vi "host_file_logging.vi"() -> ()   [LabVIEW 2011]
uses:
  Input - Cluster.ctl
  Output - Cluster.ctl
  <vilib>/Platform/TimedLoop/XDataNode/timing_clust.ctl
  <vilib>/Platform/TimedLoop/XDataNode/nitl_modes.ctl
  <vilib>/Platform/TimedLoop/XDataNode/wakeup.ctl
  <vilib>/Platform/TimedLoop/XDataNode/XDataNode.xnode
  <vilib>/Platform/TimedLoop/XDataNode/XDNodeRunTimeDep.lvlib
panel:
  in  "stop":bool
  in  "Pfad":path=path "T:/Projekt_B2G_FABES/B2G/Messprotokolle_B2G1"
  in  "Interval [s]":u32=60 min=1 step=1
  in  "Output - Cluster":T1 {"pHS-1 [pH]" format="%.2g"; "TS-4 [°C]" format="%#.2g"; "FS-2 [l]" format="%.2g"; "FS-1 [l]" format="%.2g"; "DS-1 [bar]" format="%#.2g"; "DFS-1 [l/min]" format="%#.2g"; "FS-3 [l]" format="%.2g"; "DFS-1 [l]" format="%.0g"}
  in  "File Log":bool
  in  "Input - Cluster":T2 {"P-5 AUS [min]" max=100 step=1 format="%#_3g"; "P-5 EIN [min]" step=1 format="%#_3g"; "Hysterese [°C]" format="%.1g"; "P-5 Drehzahl [%]" max=100 step=1 format="%#_3g"; "P-4 Drehzahl [%]" max=100 step=1 format="%#_3g"}
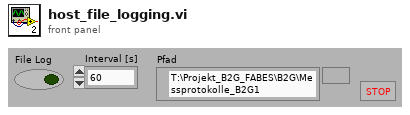
[diagram p1: front panel]
types:
  T1 = typedef "Output - Cluster.ctl" = cluster{"DFS-1 [l]":u64, "FS-3 [l]":dbl, "DFS-1 [l/min]":dbl, "DS-1 [bar]":dbl, "V-10 ZU":bool, "V-14 ZU":bool, "FS-1 [l]":dbl, "FS-2 [l]":dbl, "TS-4 [°C]":dbl, "HS-1":bool, "V-13 [%]":u8, "V-15 [%]":u8, "P-4 [%]":u8, "P-5 [%]":u8, "Dosierung":bool, "MR Max Füllstand":bool, "MR Min Füllstand":bool, "Dosiermenge [l]":sgl, "V-14 AUF":bool, "V-10 AUF":bool, "T-1 Max Füllstand":bool, "T-1 Min Füllstand":bool, "T-2 Max Füllstand":bool, "T-2 Min Füllstand":bool, "pHS-1 [pH]":dbl, "P-4":bool, "P-5":bool, "V-33 AUF":bool, "V-33 ZU":bool, "V-34 AUF":bool, "V-34 ZU":bool}
  T2 = typedef "Input - Cluster.ctl" = cluster{"V-13 [%]":u8, "V-15 [%]":u8, "Log-Target":bool, "P-4":bool, "P-4 Drehzahl [%]":u8, "Temperaturregelung":bool, "Überdruckregelung":bool, "Füllstandsregulierung":bool, "V-10":bool, "Log-Host":bool, "V-14":bool, "P-5":bool, "P-5 Drehzahl [%]":u8, "HS-1":bool, "Füllstand  P":sgl, "Füllstand I":sgl, "Füllstand D":sgl, "Füllstand Soll [l]":sgl, "Druck  P":sgl, "Druck I":sgl, "Druck D":sgl, "Druck Soll [bar]":sgl, "Temp Soll [°C]":sgl, "Dosierung":bool, "Dosiermenge [l]":sgl, "Dosiergeschw. [l/min]":sgl, "Tank":bool, "Hysterese [°C]":sgl, "MR Füllstandsüberwachung":bool, "Tank Füllstandsüberwachung":bool, "Log Target [ms]":u32, "Log Host [s]":u32, "P-5 EIN [min]":u8, "P-5 AUS [min]":u8, "Zirkulation":bool}
  T3 = typedef "XDNodeRunTimeDep.lvlib/timing_clust.ctl" = cluster{"Expected End [f-1]":u64, "Actual End [f-1]":u64, "Finished Late? [f-1]":bool, "Expected End [i-1]":u64, "Actual End [i-1]":u64, "Finished Late? [i-1]":bool, "Expected Start [i]":u64, "Actual Start [i]":u64, "Expected Start [f]":u64, "Actual Start [f]":u64, "Source Name":string, "Structure Name":string, "Period":i64, "Deadline":i64, "Offset":i64, "Start":i64, "Priority":i32, "Timeout":i32, "Mode":T4, "Wakeup Reason":T5, "Error":errorcluster, "Source Type":string, "Secondary Source Type":string, "Global End Time":u64, "Global Start Time":u64, "Frame Duration":u64, "Iteration Duration":u64, "Assigned CPU":i32, "I/O Scan Engine Mode":u32}
  T4 = typedef "XDNodeRunTimeDep.lvlib/nitl_modes.ctl" = enum32{"No Change", "Process missed periods, maintain original phase", "Discard missed periods, maintain original phase", "Process missed periods, ignore original phase", "Discard missed periods, ignore original phase"}
  T5 = typedef "XDNodeRunTimeDep.lvlib/wakeup.ctl" = enum32{"Normal", "Aborted", "Asynchronous wakeup", "Timing source error", "Timed loop error", "Timeout"}
  T6 = enum16{"open", "replace", "create", "open or create", "replace or create", "replace or create with confirmation"}
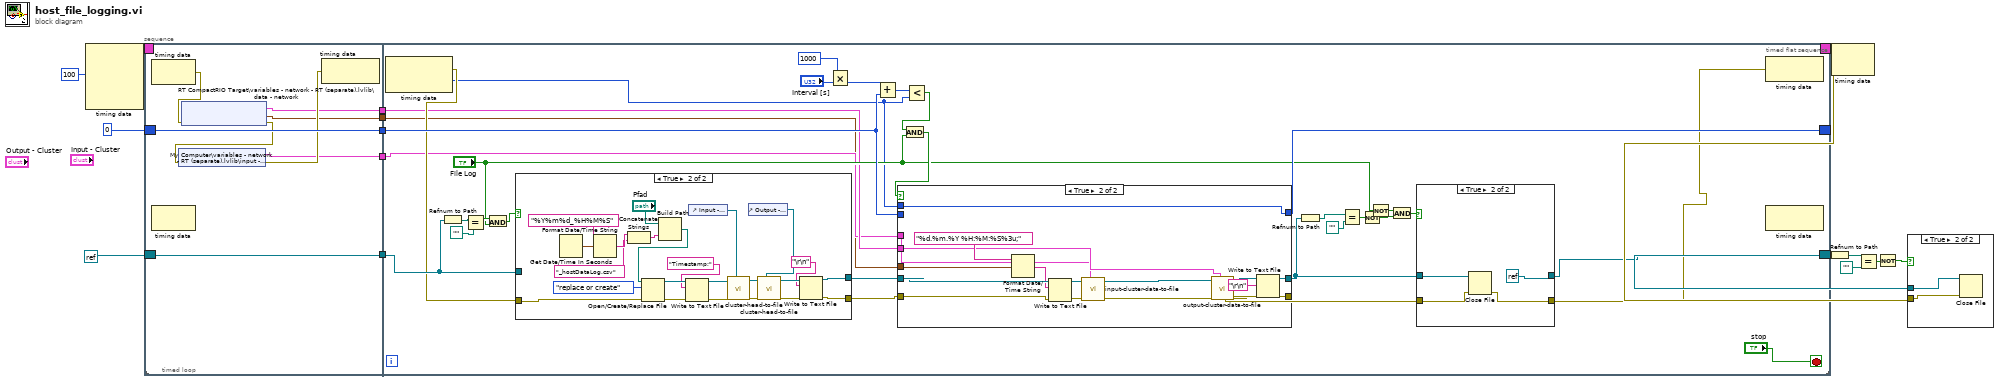
[diagram p0: block diagram]
diagram:
  n1 = node-c288(i64 100 ("Period")) -> (w11:T3)  [unwired: 3 in]
  n2 = timed-loop {
    timing: w11 -> [_]
    timing-out: [_] -> w10
    shift-right: [w14] -> w5
    shift-left: refnum<k0> refnum -> [w15]
    shift-right: [w12] -> _
    shift-left: i64 0 ("Actual Start [i]") -> [w13]
    stop <- "stop" stop-if-true
    n3 = timed-sequence {
      timing: _ -> [_]
      timing-out: _ -> [_]
      tunnel: w15 -> [w24]
      tunnel: [w23] -> w14
      tunnel: w13 -> [w22]
      tunnel: [w21] -> w12
      n4 = timed-flat-sequence {
        tunnel: w22 -> [w31]
        tunnel: w24 -> [w32]
        tunnel: [w32] -> w20
        tunnel: [w31] -> w19
        tunnel: [w27] -> w18
        tunnel: [w26] -> w17
        tunnel: [w25] -> w16
        tunnel: [w69] -> w23
        tunnel: [w51] -> w21
        tunnel: w20 -> [w53]
        tunnel: w19 -> [w50]
        tunnel: w18 -> [w41]
        tunnel: w17 -> [w40]
        tunnel: w16 -> [w39]
        frame #0 {
          n5 = node-c288() -> (w30:errorcluster)  [unwired: 1 in]
          n6 = shared-variable "RT CompactRIO Target\\variables - network - RT (separate).lvlib\\data - network"(error in=w30) -> (w27:T1, error out=w29:errorcluster, w25:timestamp)
          n7 = shared-variable "My Computer\\variables - network - RT (separate).lvlib\\input - network"(error in=w29) -> (w26:T2, error out=w28:errorcluster)
          n8 = node-c288(w28) -> ()  [unwired: 1 out]
        }
        frame #1 {
          n9 = node-c288() -> (w43:errorcluster, w38:i64)  [unwired: 1 in]
          n10 = Refnum to Path(1:w53) -> (0:w58:path)
          n11 = Equal?(x=w58, y=path "") -> (x = y?=w55:bool)
          n12 = And(x=w55, y="File Log") -> (x .and. y?=w56:bool)
          n13 = case shown="True" w56 {
            tunnel: [w90 w100] -> w59
            tunnel: [w91 w99] -> w54
            tunnel: w43 -> [w91 w92]
            tunnel: w53 -> [w90 _]
            frame False {
            }
            frame True {
              n14 = Get Date/Time In Seconds() -> (seconds since 1Jan1904=w112:timestamp)
              n15 = Format Date/Time String(time format string (%c)="%Y%m%d_%H%M%S", seconds (now)=w112) -> (date/time string=w111:string)  [unwired: 1 in]
              n16 = Concatenate Strings(w111, "_hostDataLog.csv" ("name or relative path")) -> (w108:string)
              n17 = Build Path(base path="Pfad", name or relative path=w108) -> (appended path=w107:path)
              n18 = Open/Create/Replace File(file path (use dialog)=w107, error in=w92, operation (0:open)=T6."replace or create") -> (refnum out=w97:refnum<file>, error out=w96:errorcluster)  [unwired: 3 in, 1 out]
              n19 = Write to Text File(file (use dialog)=w97, text="Timestamp;", error in=w96) -> (refnum out=w94:refnum<file>, error out=w95:errorcluster)  [unwired: 1 in, 1 out]
              n20 = control-ref of="Input - Cluster"() -> (w103:refnum<vi>)
              n21 = call "cluster-head-to-file.vi"("refnum in"=w94, "error in"=w95, "cluster ref"=w103) -> ("refnum out"=w105:refnum<file>, "error out"=w104:errorcluster)  [unwired: 6 in]
              n22 = control-ref of="Output - Cluster"() -> (w106:refnum<vi>)
              n23 = call "cluster-head-to-file.vi"("refnum in"=w105, "error in"=w104, "cluster ref"=w106) -> ("refnum out"=w102:refnum<file>, "error out"=w101:errorcluster)  [unwired: 6 in]
              n24 = Write to Text File(file (use dialog)=w102, text="\r\n", error in=w101) -> (refnum out=w100:refnum<file>, error out=w99:errorcluster)  [unwired: 1 in, 1 out]
            }
          }
          n25 = Multiply(x=u32 1000, y="Interval [s]") -> (x*y=w45:u32)
          n26 = Add(x=w45, y=w50) -> (x+y=w49:i64)
          n27 = Less?(x=w49, y=w38) -> (x < y?=w46:bool)
          n28 = And(x=w46, y="File Log") -> (x .and. y?=w48:bool)
          n29 = case shown="True" w48 {
            tunnel: [w71 w88] -> w65
            tunnel: [w72 w86] -> w67
            tunnel: w59 -> [w71 w82]
            tunnel: w54 -> [w72 w76]
            tunnel: [w70 w73] -> w51
            tunnel: w50 -> [w70 _]
            tunnel: w41 -> [_ w78]
            tunnel: w40 -> [_ w75]
            tunnel: w39 -> [_ w74]
            tunnel: w38 -> [_ w73]
            frame False {
            }
            frame True {
              n30 = Format Date/Time String(time format string (%c)="%d.%m.%Y %H:%M:%S%3u;", seconds (now)=w74) -> (date/time string=w79:string)  [unwired: 1 in]
              n31 = Write to Text File(file (use dialog)=w82, text=w79, error in=w76) -> (refnum out=w80:refnum<file>, error out=w81:errorcluster)  [unwired: 1 in, 1 out]
              n32 = call "input-cluster-data-to-file.vi"("refnum in"=w80, "error in"=w81, "Input - Cluster"=w75) -> ("refnum out"=w83:refnum<file>, "error out"=w77:errorcluster)  [unwired: 6 in]
              n33 = call "output-cluster-data-to-file.vi"("refnum in"=w83, "error in"=w77, "Output - Cluster"=w78) -> ("refnum out"=w89:refnum<file>, "error out"=w87:errorcluster)  [unwired: 6 in]
              n34 = Write to Text File(file (use dialog)=w89, text="\r\n", error in=w87) -> (refnum out=w88:refnum<file>, error out=w86:errorcluster)  [unwired: 1 in, 1 out]
            }
          }
          n35 = Refnum to Path(1:w65) -> (0:w64:path)
          n36 = Equal?(x=w64, y=path "") -> (x = y?=w62:bool)
          n37 = Not(x=w62) -> (.not. x?=w60:bool)
          n38 = Not(x="File Log") -> (.not. x?=w61:bool)
          n39 = And(x=w61, y=w60) -> (x .and. y?=w66:bool)
          n40 = case shown="True" w66 {
            tunnel: [w116 refnum<k0> refnum] -> w69
            tunnel: w65 -> [w116 w120]
            tunnel: [w115 w118] -> w42
            tunnel: w67 -> [w115 w119]
            frame False {
            }
            frame True {
              n41 = Close File(refnum=w120, error in=w119) -> (error out=w118:errorcluster)  [unwired: 1 out]
            }
          }
          n42 = node-c288(w42) -> ()  [unwired: 1 out]
        }
      }
    }
    n43 = node-c288() -> ()  [unwired: 1 in, 1 out]
    n44 = node-c288() -> ()  [unwired: 1 in, 1 out]
  }
  n45 = Refnum to Path(1:w5) -> (0:w8:path)
  n46 = node-c288(w10) -> (w1:errorcluster)
  n47 = Equal?(x=w8, y=path "") -> (x = y?=w6:bool)
  n48 = Not(x=w6) -> (.not. x?=w7:bool)
  n49 = case shown="True" w7 {
    tunnel: w5 -> [_ w130]
    tunnel: w1 -> [_ w129]
    frame False {
    }
    frame True {
      n50 = Close File(refnum=w130, error in=w129) -> ()  [unwired: 2 out]
    }
  }
